vi "Modbus Status System.vi"(0 "InterfaceData":T1 {"GenEast"."TotalFuel(L)" format="%.2f"; "GenEast"."FuelRate(L/H)" format="%.2f"; "GenEast"."ApparentPower(VA)" format="%.2f"; "GenEast"."BattVoltage(V)" format="%.2f"; "GenEast"."Freq(Hz)" format="%.2f"; "GenEast"."RunHours(hr)" format="%.2f"; "GenEast"."PowerFactor" format="%.2f"; "GenEast"."ReactivePower(VAR)" format="%.2f"; "GenEast"."ActivePower(W)" format="%.2f"; "GenWest"."TotalFuel(L)" format="%.2f"; "GenWest"."FuelRate(L/H)" format="%.2f"; "GenWest"."ApparentPower(VA)" format="%.2f"; "GenWest"."BattVoltage(V)" format="%.2f"; "GenWest"."Freq(Hz)" format="%.2f"; "GenWest"."RunHours(hr)" format="%.2f"; "GenWest"."PowerFactor" format="%.2f"; "GenWest"."ReactivePower(VAR)" format="%.2f"; "GenWest"."ActivePower(W)" format="%.2f"; "Converter Alarms 2" format="%016b"; "Converter Faults 2" format="%016b"; "Controller Faults" format="%016b"; "System Status" format="%016b"; "Converter Alarms 1" format="%016b"; "Converter Faults 1" format="%016b"; "Solar Faults" format="%016b"; "ES Rack 10 Alarms" format="%016b"; "ES Rack 9 Alarms" format="%016b"; "ES Rack 8 Alarms" format="%016b"; "ES Rack 7 Alarms" format="%016b"; "ES Rack 6 Alarms" format="%016b"; "ES Rack 5 Alarms" format="%016b"; "ES Rack 4 Alarms" format="%016b"; "ES Rack 3 Alarms" format="%016b"; "ES Rack 2 Alarms" format="%016b"; "ES Rack 1 Alarms" format="%016b"; "ES System Alarms" format="%016b"; "System Faults" format="%016b"; "ES Rack 10 Faults" format="%016b"; "ES Rack 9 Faults" format="%016b"; "ES Rack 8 Faults" format="%016b"; "ES Rack 7  Faults" format="%016b"; "ES Rack 6 Faults" format="%016b"; "ES Rack 5 Faults" format="%016b"; "ES Rack 4 Faults" format="%016b"; "ES Rack 3 Faults" format="%016b"; "ES Rack 2 Faults" format="%016b"; "ES Rack 1 Faults" format="%016b"; "ES System Faults" format="%016b"}, 1 "ES System Data In":T7={"Voltage"=0.0, "Current"=0.0, "SOC Avg"=0.0, "Faults"=0, "Alarms"=0, "# Strings"=0, "Max Temp"=0, "Min Temp"=0, "Max Cell Voltage"=0.0, "Min Cell Voltage"=0.0, "Energy Capacity"=0.0, "Energy Remaining"=0.0, "SOC Min"=0.0, "SOC Max"=0.0, "ES Fault"=FALSE, "String Select"=enum."3 Strings", "ES Com Fault"=FALSE, "SOH Avg"=0.0}, 3 "Gen Data Array":T2[](array[typedef]) {"TotalFuel(L)" format="%.2f"; "FuelRate(L/H)" format="%.2f"; "ApparentPower(VA)" format="%.2f"; "BattVoltage(V)" format="%.2f"; "Freq(Hz)" format="%.2f"; "RunHours(hr)" format="%.2f"; "PowerFactor" format="%.2f"; "ReactivePower(VAR)" format="%.2f"; "ActivePower(W)" format="%.2f"}, 5 "PC Data In":T5 {"Alarms 2" format="%016b"; "Faults 2" format="%016b"; "Alarms 1" format="%016b"; "Faults 1" format="%016b"; "Contactor FB" format="%.0b"; "DC Voltage SP" format="%2.1f"; "Clear Faults SP" format="%.0b"; "Neutral Current" format="%2.1f"; "AC Current - L2" format="%2.1f"; "AC Voltage - L2" format="%2.1f"; "Temperature" format="%2.1f"; "DC Voltage" format="%2.1f"; "AC Current SP" format="%2.1f"; "AC Voltage SP" format="%2.1f"; "Frequency SP" format="%2.1f"; "AC Frequency" format="%2.1f"; "AC Current - L1" format="%2.1f"; "AC Voltage- L1" format="%2.1f"}, 7 "isGenOn":bool[](array[boolean]), 9 "FPGA Data In":T4 {"SSG Active Current" format="%2.1f"; "PV Reactive Power (L1)" format="%2.1f"; "PV Reactive Power (L2)" format="%2.1f"; "PV Total Reactive Power" format="%2.1f"; "Gen Reactive Power (L1)" format="%2.1f"; "Gen Reactive Power (L2)" format="%2.1f"; "Gen Total Reactive Power" format="%2.1f"; "SSG Reactive Power (L1)" format="%2.1f"; "SSG Reactive Power (L2)" format="%2.1f"; "SSG Total Reactive Power" format="%2.1f"; "PV Total Current" format="%2.1f"; "PV Total Voltage" format="%2.1f"; "PV Active Power (L1)" format="%2.1f"; "PV Active Power (L2)" format="%2.1f"; "PV App Power (L1)" format="%2.1f"; "PV App Power (L2)" format="%2.1f"; "PV Total Active Power" format="%2.1f"; "PV Total App Power" format="%2.1f"; "PV Arms (L1)" format="%2.1f"; "PV Arms (L2)" format="%2.1f"; "PV Vrms (L1)" format="%2.1f"; "PV Vrms (L2)" format="%2.1f"; "Gen Total Current" format="%2.1f"; "SSG Total Current" format="%2.1f"; "Gen Total Voltage" format="%2.1f"; "SSG Total Voltage" format="%2.1f"; "Gen Active Power (L1)" format="%2.1f"; "Gen Active Power (L2)" format="%2.1f"; "SSG Active Power (L1)" format="%2.1f"; "SSG Active Power (L2)" format="%2.1f"; "Gen App Power (L1)" format="%2.1f"; "Gen App Power (L2)" format="%2.1f"; "SSG App Power (L1)" format="%2.1f"; "SSG App Power (L2)" format="%2.1f"; "Gen Total Active Power" format="%2.1f"; "Gen Total App Power" format="%2.1f"; "Gen Arms (L1)" format="%2.1f"; "Gen Arms (L2)" format="%2.1f"; "Gen Vrms (L1)" format="%2.1f"; "Gen Vrms (L2)" format="%2.1f"; "SSG Total Active Power" format="%2.1f"; "SSG Total App Power" format="%2.1f"; "SSG Arms (L1)" format="%2.1f"; "SSG Arms (L2)" format="%2.1f"; "SSG Vrms (L1)" format="%2.1f"; "SSG Vrms (L2)" format="%2.1f"}, 11 "Error In":errorcluster, 12 "Real Time State":T3, 13 "Manual Shutdown":bool=TRUE, 14 "Gen Start Fault":bool=TRUE) -> (4 "InterfaceData":T1 {"GenEast"."TotalFuel(L)" format="%.2f"; "GenEast"."FuelRate(L/H)" format="%.2f"; "GenEast"."ApparentPower(VA)" format="%.2f"; "GenEast"."BattVoltage(V)" format="%.2f"; "GenEast"."Freq(Hz)" format="%.2f"; "GenEast"."RunHours(hr)" format="%.2f"; "GenEast"."PowerFactor" format="%.2f"; "GenEast"."ReactivePower(VAR)" format="%.2f"; "GenEast"."ActivePower(W)" format="%.2f"; "GenWest"."TotalFuel(L)" format="%.2f"; "GenWest"."FuelRate(L/H)" format="%.2f"; "GenWest"."ApparentPower(VA)" format="%.2f"; "GenWest"."BattVoltage(V)" format="%.2f"; "GenWest"."Freq(Hz)" format="%.2f"; "GenWest"."RunHours(hr)" format="%.2f"; "GenWest"."PowerFactor" format="%.2f"; "GenWest"."ReactivePower(VAR)" format="%.2f"; "GenWest"."ActivePower(W)" format="%.2f"; "Converter Alarms 2" format="%016b"; "Converter Faults 2" format="%016b"; "Controller Faults" format="%016b"; "System Status" format="%016b"; "Converter Alarms 1" format="%016b"; "Converter Faults 1" format="%016b"; "Solar Faults" format="%016b"; "ES Rack 10 Alarms" format="%016b"; "ES Rack 9 Alarms" format="%016b"; "ES Rack 8 Alarms" format="%016b"; "ES Rack 7 Alarms" format="%016b"; "ES Rack 6 Alarms" format="%016b"; "ES Rack 5 Alarms" format="%016b"; "ES Rack 4 Alarms" format="%016b"; "ES Rack 3 Alarms" format="%016b"; "ES Rack 2 Alarms" format="%016b"; "ES Rack 1 Alarms" format="%016b"; "ES System Alarms" format="%016b"; "System Faults" format="%016b"; "ES Rack 10 Faults" format="%016b"; "ES Rack 9 Faults" format="%016b"; "ES Rack 8 Faults" format="%016b"; "ES Rack 7  Faults" format="%016b"; "ES Rack 6 Faults" format="%016b"; "ES Rack 5 Faults" format="%016b"; "ES Rack 4 Faults" format="%016b"; "ES Rack 3 Faults" format="%016b"; "ES Rack 2 Faults" format="%016b"; "ES Rack 1 Faults" format="%016b"; "ES System Faults" format="%016b"}, 15 "Error Out":errorcluster)   [LabVIEW 2014]
uses:
  Controls/ES System Data.ctl
  Controls/StringSelector.ctl
  Controls/PC Data.ctl
  Controls/MicroZed Config Op Mode.ctl
  Controls/FPGA Data.ctl
  Controls/Gen Data.ctl
  Controls/RT State.ctl
  Controls/Interface Data.ctl
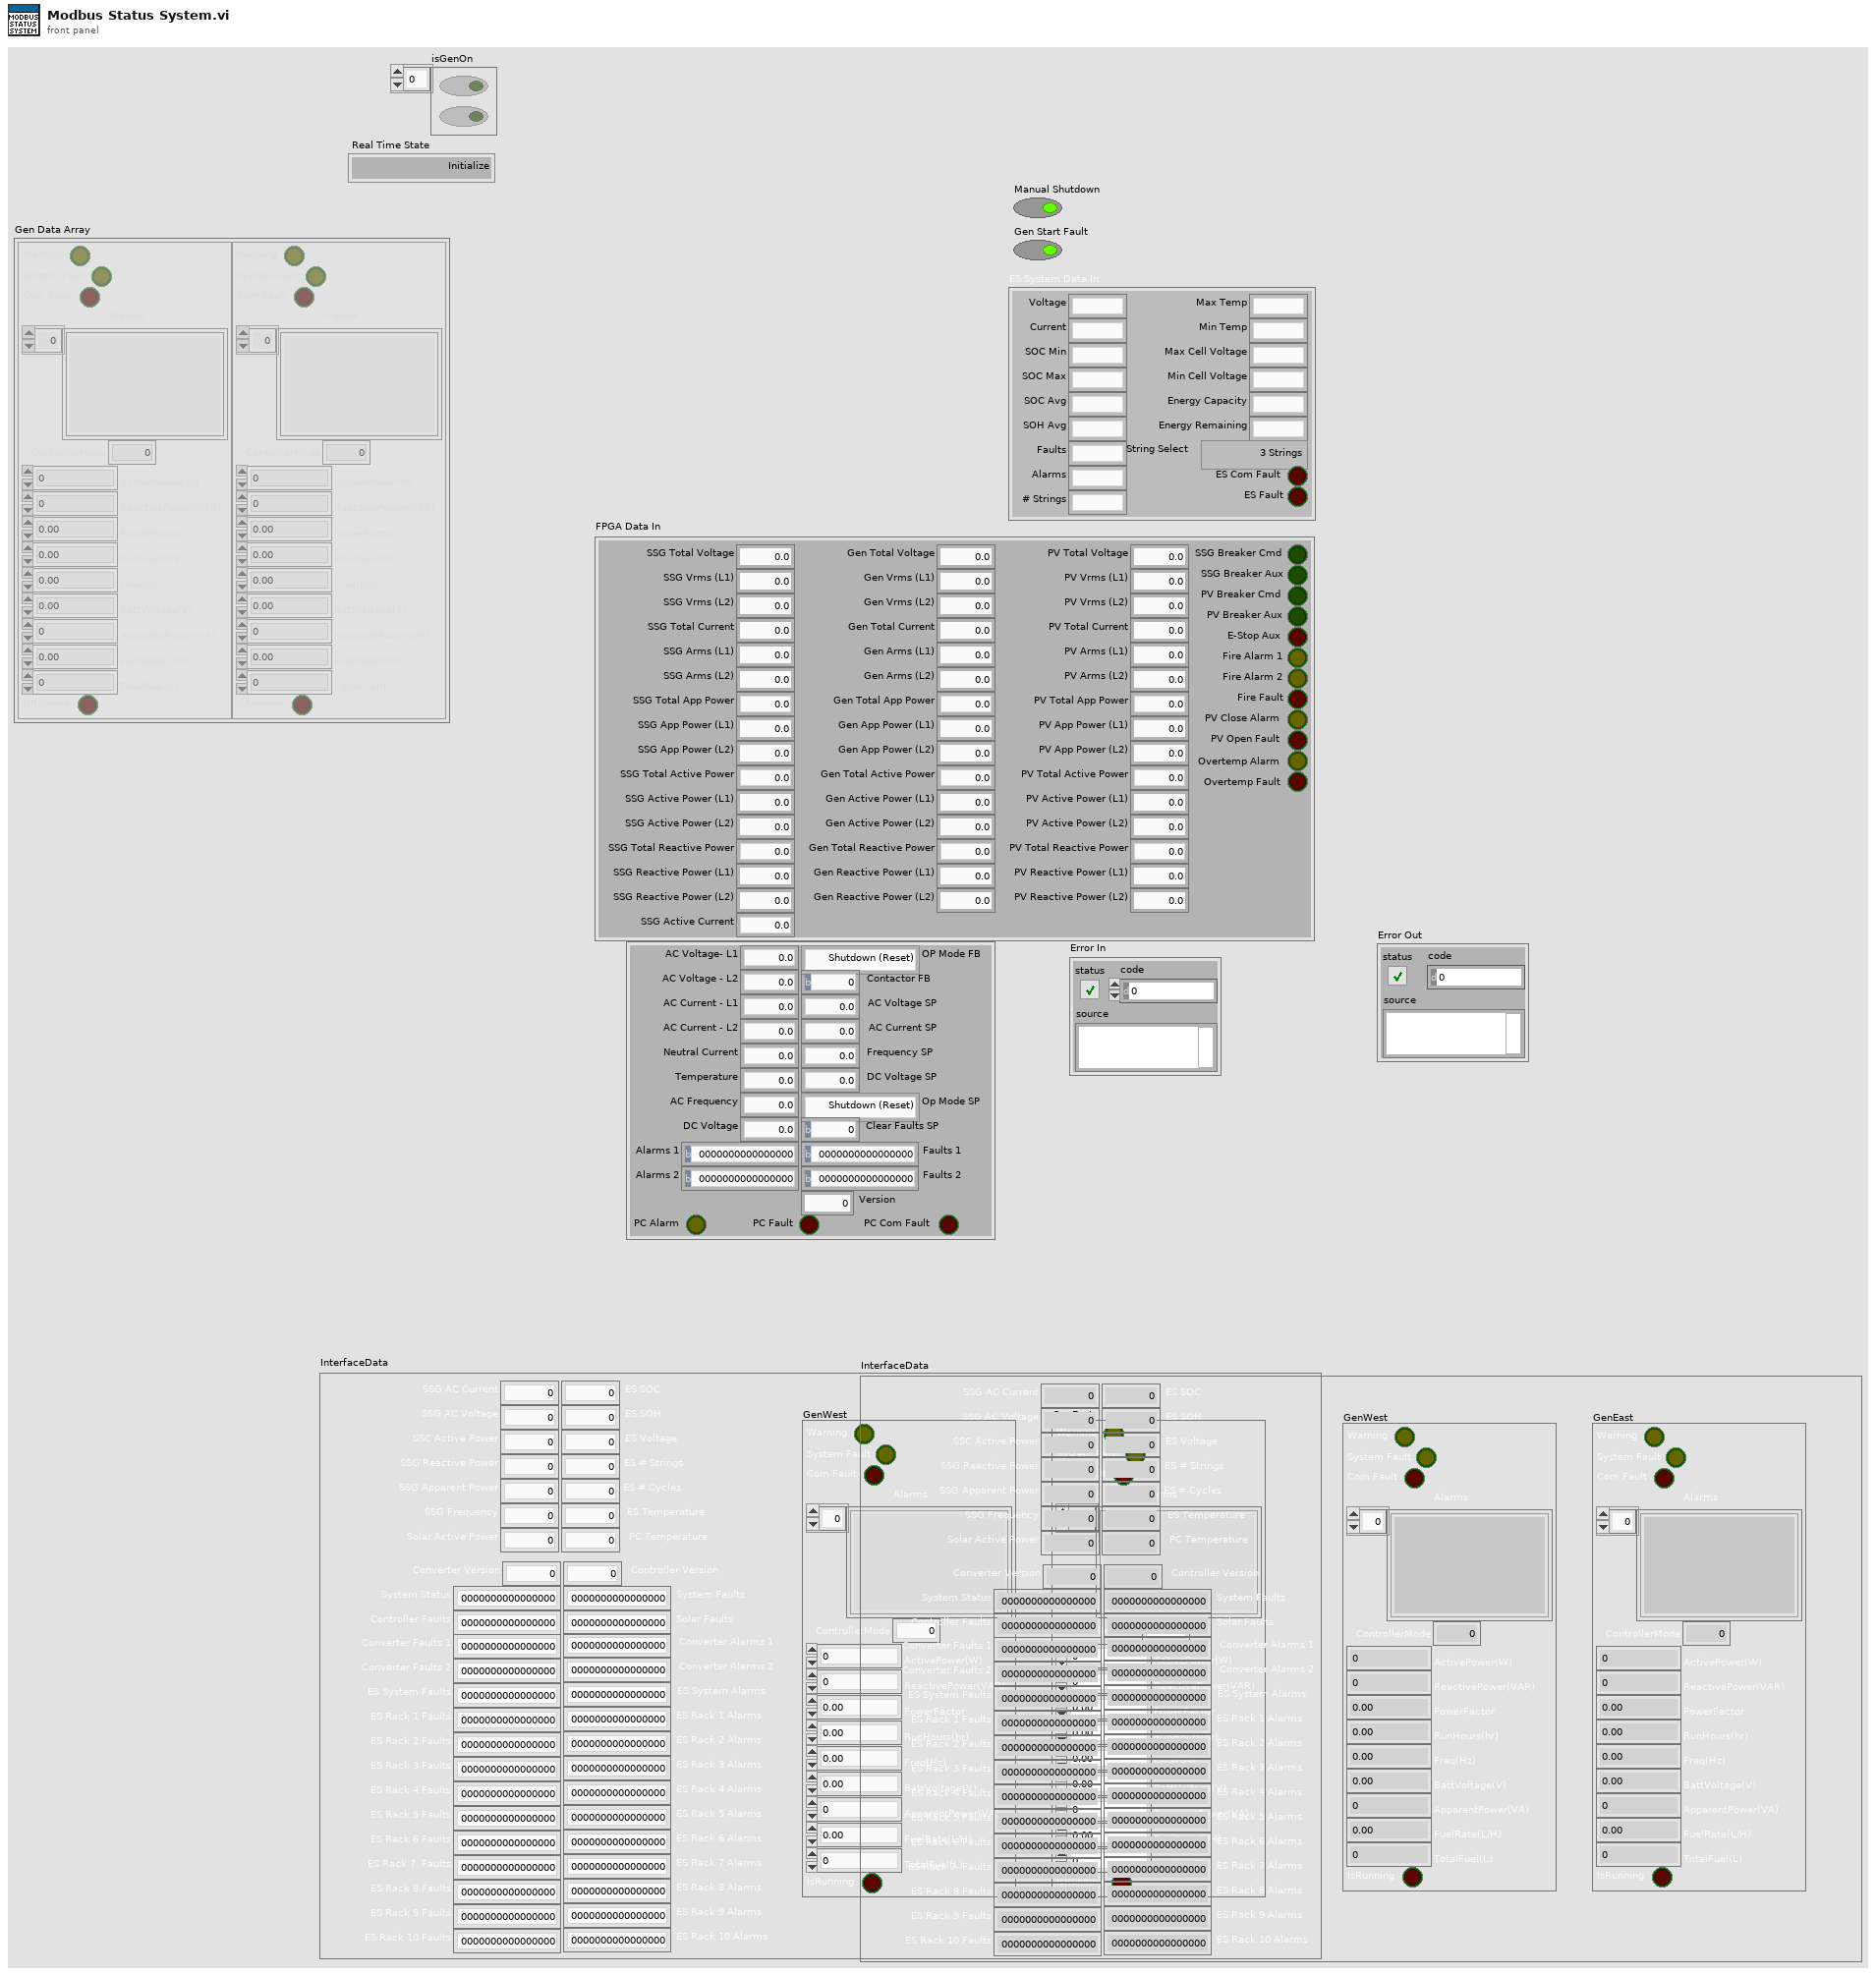
[diagram p1: front panel]
types:
  T1 = typedef "Interface Data.ctl" = cluster{"SSG AC Current":i16, "SSG AC Voltage":i16, "SSC Active Power":i16, "SSG Reactive Power":i16, "SSG Apparent Power":i16, "SSG Frequency":i16, "ES SOC":i16, "ES SOH":i16, "ES Voltage":i16, "ES # Strings":i16, "ES # Cycles":i16, "ES Temperature":i16, "PC Temperature":i16, "Solar Active Power":i16, "Converter Version":i16, "Controller Version":i16, "System Status":i16, "System Faults":i16, "Controller Faults":i16, "ES System Faults":i16, "ES System Alarms":i16, "Converter Faults 1":i16, "Converter Faults 2":i16, "Converter Alarms 1":i16, "Converter Alarms 2":i16, "Solar Faults":i16, "ES Rack 1 Faults":i16, "ES Rack 2 Faults":i16, "ES Rack 3 Faults":i16, "ES Rack 4 Faults":i16, "ES Rack 5 Faults":i16, "ES Rack 6 Faults":i16, "ES Rack 7  Faults":i16, "ES Rack 8 Faults":i16, "ES Rack 9 Faults":i16, "ES Rack 10 Faults":i16, "ES Rack 1 Alarms":i16, "ES Rack 2 Alarms":i16, "ES Rack 3 Alarms":i16, "ES Rack 4 Alarms":i16, "ES Rack 5 Alarms":i16, "ES Rack 6 Alarms":i16, "ES Rack 7 Alarms":i16, "ES Rack 8 Alarms":i16, "ES Rack 9 Alarms":i16, "ES Rack 10 Alarms":i16, "GenWest":T2, "GenEast":T2}
  T2 = typedef "Gen Data.ctl" = cluster{"Warning":bool, "System Fault":bool, "Com Fault":bool, "Alarms":string[], "ControllerMode":u16, "ActivePower(W)":i32, "ReactivePower(VAR)":i32, "PowerFactor":dbl, "RunHours(hr)":dbl, "Freq(Hz)":dbl, "BattVoltage(V)":dbl, "ApparentPower(VA)":i32, "FuelRate(L/H)":dbl, "TotalFuel(L)":u32, "IsRunning":bool}
  T3 = typedef "RT State.ctl" = enum16{"Initialize", "Ready", "Startup 1 - Start Genset", "Startup 2 - Start Inverter", "Startup 3 - Battery Match", "SpotGen - Start", "SpotGen - Charge", "SpotGen - Desync", "SpotGen - Discharge", "SpotGen - Sync", "Shutdown", "INVALID STATE"}
  T4 = typedef "FPGA Data.ctl" = cluster{"Gen Total Voltage":dbl, "Gen Vrms (L1)":dbl, "Gen Vrms (L2)":dbl, "Gen Total Current":dbl, "Gen Arms (L1)":dbl, "Gen Arms (L2)":dbl, "Gen Total App Power":dbl, "Gen App Power (L1)":dbl, "Gen App Power (L2)":dbl, "Gen Total Active Power":dbl, "Gen Active Power (L1)":dbl, "Gen Active Power (L2)":dbl, "Gen Total Reactive Power":dbl, "Gen Reactive Power (L1)":dbl, "Gen Reactive Power (L2)":dbl, "SSG Total Voltage":dbl, "SSG Vrms (L1)":dbl, "SSG Vrms (L2)":dbl, "SSG Total Current":dbl, "SSG Arms (L1)":dbl, "SSG Arms (L2)":dbl, "SSG Total App Power":dbl, "SSG App Power (L1)":dbl, "SSG App Power (L2)":dbl, "SSG Total Active Power":dbl, "SSG Active Power (L1)":dbl, "SSG Active Power (L2)":dbl, "SSG Total Reactive Power":dbl, "SSG Reactive Power (L1)":dbl, "SSG Reactive Power (L2)":dbl, "PV Total Voltage":dbl, "PV Vrms (L1)":dbl, "PV Vrms (L2)":dbl, "PV Total Current":dbl, "PV Arms (L1)":dbl, "PV Arms (L2)":dbl, "PV Total App Power":dbl, "PV App Power (L1)":dbl, "PV App Power (L2)":dbl, "PV Total Active Power":dbl, "PV Active Power (L1)":dbl, "PV Active Power (L2)":dbl, "PV Total Reactive Power":dbl, "PV Reactive Power (L1)":dbl, "PV Reactive Power (L2)":dbl, "SSG Breaker Cmd":bool, "SSG Breaker Aux":bool, "PV Breaker Cmd":bool, "PV Breaker Aux":bool, "E-Stop Aux":bool, "Fire Alarm 1":bool, "Fire Alarm 2":bool, "Fire Fault":bool, "PV Close Alarm":bool, "SSG Active Current":dbl, "Overtemp Alarm":bool, "Overtemp Fault":bool, "PV Open Fault":bool}
  T5 = typedef "PC Data.ctl" = cluster{"AC Voltage- L1":dbl, "AC Voltage - L2":dbl, "AC Current - L1":dbl, "AC Current - L2":dbl, "Neutral Current":dbl, "Temperature":dbl, "AC Frequency":dbl, "DC Voltage":dbl, "AC Voltage SP":dbl, "AC Current SP":dbl, "Frequency SP":dbl, "Op Mode SP":T6, "Clear Faults SP":u16, "PC Com Fault":bool, "PC Fault":bool, "DC Voltage SP":dbl, "OP Mode FB":T6, "Contactor FB":u16, "Faults 1":u16, "Alarms 1":u16, "Faults 2":u16, "Alarms 2":u16, "PC Alarm":bool, "Version":u16}
  T6 = typedef "MicroZed Config Op Mode.ctl" = enum16{"Shutdown (Reset)", "Startup", "Idle", "Voltage Mode", "Current Mode", "Fault", "OL Voltage (Debug)", "No Data"}
  T7 = typedef "ES System Data.ctl" = cluster{"Voltage":sgl, "Current":sgl, "SOC Avg":sgl, "Faults":u16, "Alarms":u16, "# Strings":u16, "Max Temp":i16, "Min Temp":i16, "Max Cell Voltage":sgl, "Min Cell Voltage":sgl, "Energy Capacity":sgl, "Energy Remaining":sgl, "SOC Min":sgl, "SOC Max":sgl, "ES Fault":bool, "String Select":T8, "ES Com Fault":bool, "SOH Avg":sgl}
  T8 = typedef "StringSelector.ctl" = enum16{"1 String (1)", "1 String (2)", "1 String (3)", "2 Strings (1 2)", "2 Strings (2 3)", "2 Strings (1 3)", "3 Strings"}
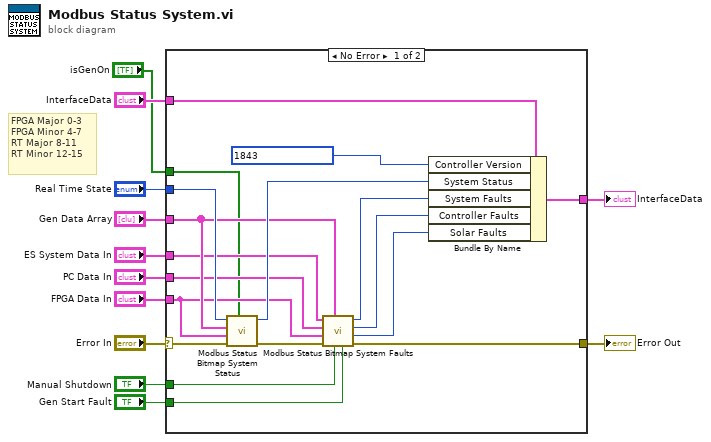
[diagram p0: block diagram]
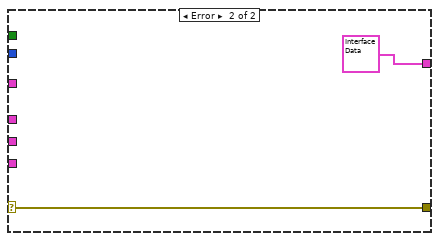
[diagram p2: hidden frame]
diagram:
  # "FPGA Major 0-3\nFPGA Minor 4-7\nRT Major 8-11\nRT Minor 12-15"
  n1 = case shown="No Error" "Error In" {
    selector: "Error In" -> [w28 w32]
    tunnel: "Gen Data Array" -> [w21 _]
    tunnel: "FPGA Data In" -> [w18 _]
    tunnel: [w24 w32] -> w9
    tunnel: "InterfaceData" -> [w30 _]
    tunnel: [w29 T1 {"SSG AC Current"=0, "SSG AC Voltage"=0, "SSC Active Power"=0, "SSG Reactive Power"=0, "SSG Apparent Power"=0, "SSG Frequency"=0, "ES SOC"=0, "ES SOH"=0, "ES Voltage"=0, "ES # Strings"=0, "ES # Cycles"=0, "ES Temperature"=0, "PC Temperature"=0, "Solar Active Power"=0, "Converter Version"=0, "Controller Version"=0, "System Status"=0, "System Faults"=0, "Controller Faults"=0, "ES System Faults"=0, "ES System Alarms"=0, "Converter Faults 1"=0, "Converter Faults 2"=0, "Converter Alarms 1"=0, "Converter Alarms 2"=0, "Solar Faults"=0, "ES Rack 1 Faults"=0, "ES Rack 2 Faults"=0, "ES Rack 3 Faults"=0, "ES Rack 4 Faults"=0, "ES Rack 5 Faults"=0, "ES Rack 6 Faults"=0, "ES Rack 7  Faults"=0, "ES Rack 8 Faults"=0, "ES Rack 9 Faults"=0, "ES Rack 10 Faults"=0, "ES Rack 1 Alarms"=0, "ES Rack 2 Alarms"=0, "ES Rack 3 Alarms"=0, "ES Rack 4 Alarms"=0, "ES Rack 5 Alarms"=0, "ES Rack 6 Alarms"=0, "ES Rack 7 Alarms"=0, "ES Rack 8 Alarms"=0, "ES Rack 9 Alarms"=0, "ES Rack 10 Alarms"=0, "GenWest"={"Warning"=FALSE, "System Fault"=FALSE, "Com Fault"=FALSE, "Alarms"=[], "ControllerMode"=0, "ActivePower(W)"=0, "ReactivePower(VAR)"=0, "PowerFactor"=0.0, "RunHours(hr)"=0.0, "Freq(Hz)"=0.0, "BattVoltage(V)"=0.0, "ApparentPower(VA)"=0, "FuelRate(L/H)"=0.0, "TotalFuel(L)"=0, "IsRunning"=FALSE}, "GenEast"={"Warning"=FALSE, "System Fault"=FALSE, "Com Fault"=FALSE, "Alarms"=[], "ControllerMode"=0, "ActivePower(W)"=0, "ReactivePower(VAR)"=0, "PowerFactor"=0.0, "RunHours(hr)"=0.0, "Freq(Hz)"=0.0, "BattVoltage(V)"=0.0, "ApparentPower(VA)"=0, "FuelRate(L/H)"=0.0, "TotalFuel(L)"=0, "IsRunning"=FALSE}} ("Modbus Status Interface Data Out")] -> w7
    tunnel: "Real Time State" -> [w27 _]
    tunnel: "ES System Data In" -> [w20 _]
    tunnel: "PC Data In" -> [w19 _]
    tunnel: "Manual Shutdown" -> [w15 _]
    tunnel: "Gen Start Fault" -> [w14 _]
    tunnel: "isGenOn" -> [w13 _]
    frame No Error {
      n2 = call "Modbus Status Bitmap System Status.vi"("isGenOn"=w13, "Error In"=w28, "FPGA Data In"=w18, "Gen Data Array"=w21, "Real Time State"=w27) -> ("Error Out"=w25:errorcluster, "System Status"=w26:i16)  [unwired: 5 in]
      n3 = call "Modbus Status Bitmap System Faults.vi"("Gen Start Fault"=w14, "Manual Shutdown"=w15, "Gen Data Array"=w21, "Error In"=w25, "FPGA Data In"=w18, "PC Data In"=w19, "ES System Data In"=w20) -> ("Error Out"=w24:errorcluster, "PV Faults"=w17:i16, "Controller Faults"=w22:i16, "System Faults"=w23:i16)  [unwired: 1 in]
      n4 = Bundle By Name(cluster=w30, "Controller Version"=i16 1843, "System Status"=w26, "System Faults"=w23, "Controller Faults"=w22, "Solar Faults"=w17) -> (w29:T1)
    }
    frame Error {
    }
  }
  "Error Out" <- w9
  "InterfaceData" <- w7
